vi "locate diagnostic set.vi"(8 "guess index":i32, 10 "device":u8, 11 "diagnostics":T1[](array[typedef])) -> (2 "found?":bool, 3 "index":i32)   [LabVIEW 2013, in "Profibus Module runtime.lvclass"]
uses:
  Profibus Module runtime.lvclass
  profibus diagnostics reporting.ctl
  configuration/error throw specification.ctl
  configuration/Profibus Module configuration.lvclass
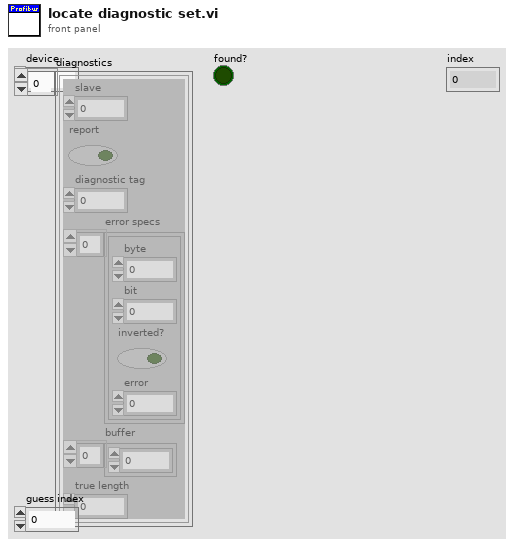
[diagram p1: front panel]
types:
  T1 = typedef "Profibus Module runtime.lvclass/profibus diagnostics reporting.ctl" = cluster{"slave":i8, "report":bool, "diagnostic tag":i32, "error specs":T2[], "buffer":u8[], "true length":u8}
  T2 = typedef "Profibus Module configuration.lvclass/error throw specification.ctl" = cluster{"byte":i32, "bit":i32, "inverted?":bool, "error":i32}
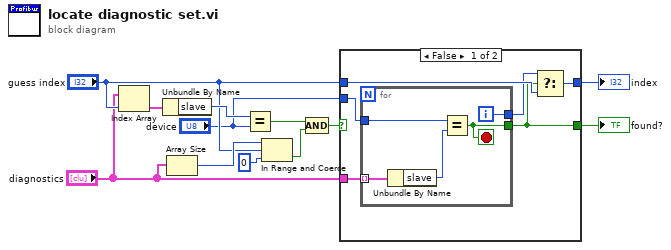
[diagram p0: block diagram]
diagram:
  n1 = Index Array(array="diagnostics", index="guess index") -> (element=w12:T1)
  n2 = Unbundle By Name(w12) -> ("slave"=w11:i8)
  n3 = Array Size(array="diagnostics") -> (size(s)=w9:i32)
  n4 = Equal?(x=w11, y="device") -> (x = y?=w10:bool)
  n5 = In Range and Coerce(upper limit=w9, x="guess index", lower limit=0) -> (In Range?=w7:bool)  [unwired: 1 out]
  n6 = Compound Arithmetic op=AND(w10, w7) -> (w6:bool)
  n7 = case shown="False" w6 {
    selector: w6 -> [_ w24]
    tunnel: [w14 w25] -> w1
    tunnel: "device" -> [w18 _]
    tunnel: "guess index" -> [w16 w25]
    tunnel: "diagnostics" -> [w17 _]
    tunnel: [w13 w24] -> w2
    frame False {
      n8 = for {
        tunnel: w17 -> [w23] mode=indexing
        tunnel: w18 -> [w21]
        tunnel: [w20] -> w15
        tunnel: [w19] -> w13
        i -> [w20]
        stop <- w19 stop-if-true
        n9 = Unbundle By Name(w23) -> ("slave"=w22:i8)
        n10 = Equal?(x=w21, y=w22) -> (x = y?=w19:bool)
      }
      n11 = Select(t=w15, s=w13, f=w16) -> (s? t:f=w14:i32)
    }
    frame True {
    }
  }
  "found?" <- w2
  "index" <- w1
